vi "Set Write Enabled.vi"(8 "error in":errorcluster, 11 "PPT in":refnum<class "PPT.lvclass">) -> (0 "error out":errorcluster, 3 "PPT out":refnum<class "PPT.lvclass">)   [LabVIEW 2014, in "PPT.lvclass"]
uses:
  PPT.lvclass
  Reusable/Session APIs/Text Communication/Text Device Session.lvclass
  PPT.lvclass/PPT.ctl
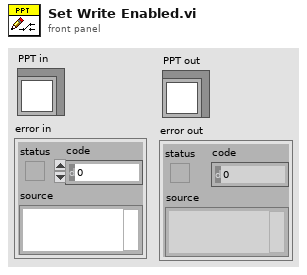
[diagram p1: front panel]
types:
  T1 = typedef "Session - Root.lvclass/Session Handle.ctl" = refnum<data-value>
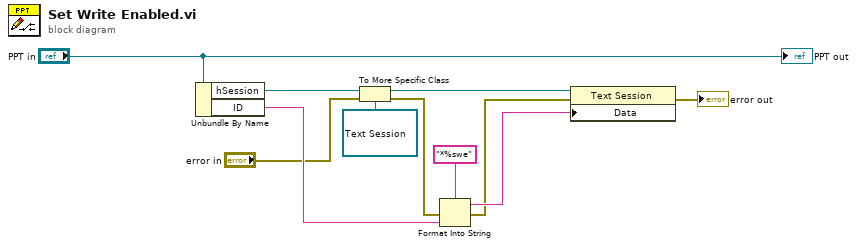
[diagram p0: block diagram]
diagram:
  n1 = Unbundle By Name("PPT in") -> ("hSession"=w10:T1, "ID"=w6:string)
  n2 = To More Specific Class(target class=refnum<data-value> refnum ("hSession"), reference=w10, error in="error in") -> (specific class reference=w8:refnum<data-value>, error out=w1:errorcluster)
  n3 = Format Into String(format string="*%swe", error in=w1, w6) -> (resulting string=w5:string, error out=w4:errorcluster)  [unwired: 1 in]
  n4 = property class="Text Session"(reference=w8, error in=w4, "Data"=w5) -> (error out=→"error out":errorcluster)  [unwired: 1 out]
  "PPT out" <- "PPT in"
